vi "pic_JudgeMotion.vi"(0 "CmdLib In":refnum<k24>, 1 "右？":bool, 5 "Llimit":bool, 7 "Motor":i32, 9 "Rlimit":bool, 11 "error in (no error)":errorcluster, 12 "零位？":bool) -> (4 "CmdLib Out":refnum<k24>, 15 "error out":errorcluster)   [LabVIEW 2018]
uses:
  Device VIs/CmdLib.dll
  Device VIs/Verbal.vi
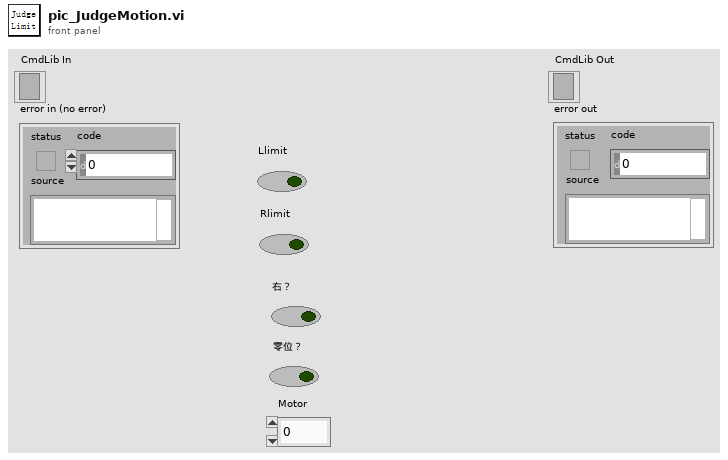
[diagram p1: front panel]
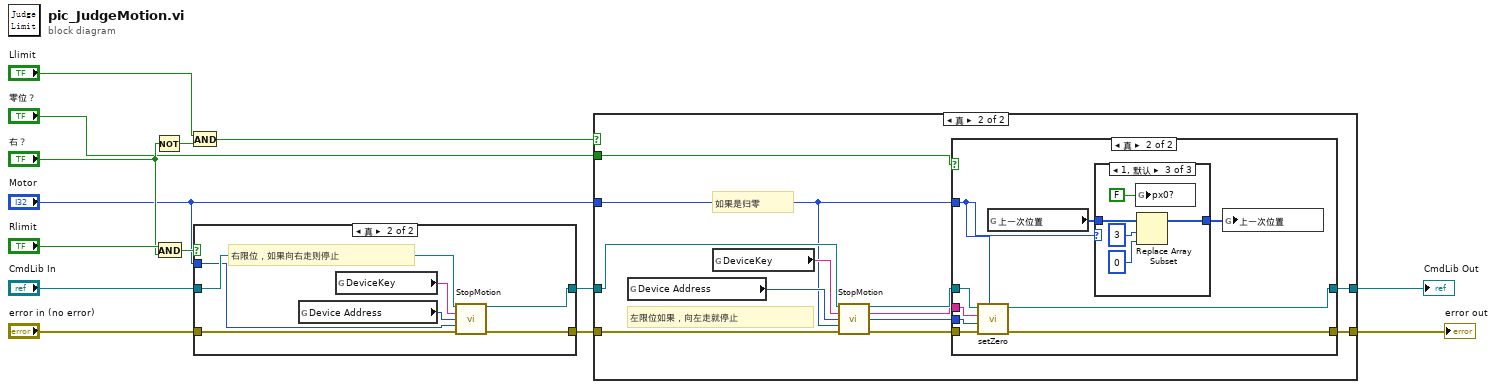
[diagram p0: block diagram]
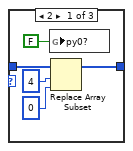
[diagram p5: hidden frame]
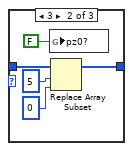
[diagram p6: hidden frame]
diagram:
  n1 = Not(x="右？") -> (.not. x?=w6:bool)
  n2 = And(x="Rlimit", y="右？") -> (x .and. y?=w9:bool)
  n3 = And(x="Llimit", y=w6) -> (x .and. y?=w13:bool)
  n4 = case shown="真" w9 {
    tunnel: "CmdLib In" -> [w16 w23]
    tunnel: "error in (no error)" -> [w15 w20]
    tunnel: [w16 w22] -> w3
    tunnel: [w15 w21] -> w2
    tunnel: "Motor" -> [_ w17]
    frame False {
    }
    frame True {
      # "右限位，如果向右走则停止"
      n5 = global read "Verbal.vi" "Device Address"() -> (w18:i32)
      n6 = global read "Verbal.vi" "DeviceKey"() -> (w19:string)
      n7 = call "StopMotion.vi"("CmdLib In"=w23, "DeviceKey In"=w19, "Device Address In"=w18, "Motor"=w17, "error in (no error)"=w20) -> ("CmdLib Out"=w22:refnum<k24>, "error out"=w21:errorcluster)  [unwired: 7 in, 2 out]
    }
  }
  n8 = case shown="真" w13 {
    tunnel: w2 -> [w24 w30]
    tunnel: w3 -> [w25 w34]
    tunnel: [w25 w36] -> w12
    tunnel: [w24 w35] -> w11
    tunnel: "零位？" -> [_ w37]
    tunnel: "Motor" -> [_ w31]
    frame False {
    }
    frame True {
      # "如果是归零"
      # "左限位如果，向左走就停止"
      n9 = global read "Verbal.vi" "Device Address"() -> (w32:i32)
      n10 = global read "Verbal.vi" "DeviceKey"() -> (w33:string)
      n11 = call "StopMotion.vi"("CmdLib In"=w34, "DeviceKey In"=w33, "Device Address In"=w32, "Motor"=w31, "error in (no error)"=w30) -> ("CmdLib Out"=w29:refnum<k24>, "DeviceKey Out"=w28:string, "Device Address Out"=w27:i32, "error out"=w26:errorcluster)  [unwired: 7 in]
      n12 = case shown="真" w37 {
        tunnel: w31 -> [_ w44]
        tunnel: [w39 w43] -> w36
        tunnel: [w38 w42] -> w35
        tunnel: w29 -> [w39 w48]
        tunnel: w28 -> [_ w47]
        tunnel: w27 -> [_ w46]
        tunnel: w26 -> [w38 w45]
        frame False {
        }
        frame True {
          n13 = call "setZero.vi"("Motor"=w44, "error in (no error)"=w45, "Device Address In"=w46, "DeviceKey In"=w47, "CmdLib In"=w48) -> ("error out"=w42:errorcluster, "CmdLib Out"=w43:refnum<k24>)  [unwired: 3 in, 2 out]
          n14 = global read "Verbal.vi" "上一次位置"() -> (w41:i32[])
          n15 = case shown="1, 默认" w44 {
            tunnel: w41 -> [w50 w55 w60]
            tunnel: [w49 w54 w59] -> w40
            frame 2 {
              n16 = global write "Verbal.vi" "py0?"(FALSE) -> ()
              n17 = Replace Array Subset(array=w50, new element=0 ("新元素/子数组"), index=4 ("索引")) -> (w49:i32[])
            }
            frame 3 {
              n18 = global write "Verbal.vi" "pz0?"(FALSE ("pz0?")) -> ()
              n19 = Replace Array Subset(array=w55, new element=0 ("新元素/子数组"), index=5 ("索引")) -> (w54:i32[])
            }
            frame 1, Default {
              n20 = global write "Verbal.vi" "px0?"(FALSE) -> ()
              n21 = Replace Array Subset(array=w60, new element=0 ("新元素/子数组"), index=3 ("索引")) -> (w59:i32[])
            }
          }
          n22 = global write "Verbal.vi" "上一次位置"(w40) -> ()
        }
      }
    }
  }
  "CmdLib Out" <- w12
  "error out" <- w11
